vi "Magnitude Coerce.vi"(8 "Magnitude Limit":dbl, 11 "x":dbl) -> (0 "In Range?":bool, 3 "Coerce(x)":dbl)   [LabVIEW 2011]
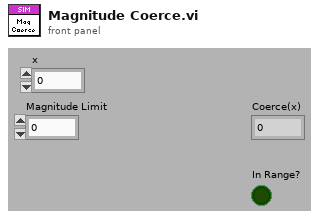
[diagram p1: front panel]
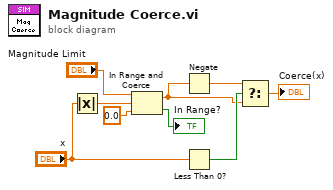
[diagram p0: block diagram]
diagram:
  n1 = Absolute Value(x="x") -> (abs(x)=w8:dbl)
  n2 = In Range and Coerce(upper limit="Magnitude Limit", x=w8, lower limit=0.0) -> (coerced(x)=w2:dbl, In Range?=→"In Range?":bool)
  n3 = Negate(x=w2) -> (-x=w3:dbl)
  n4 = Less Than 0?(x="x") -> (x < 0?=w5:bool)
  n5 = Select(t=w3, s=w5, f=w2) -> (s? t:f=→"Coerce(x)":dbl)
